vi "StandAloneTransient_TestBenchParametersArrayCreation.vi"(0 "Input Voltage Array":string[](array[string]), 1 "Board Number":string, 2 "DUT":string, 3 "Nominal Current (A)":string, 4 "XINC":string, 5 "Test Type":string, 6 "Effective LET":string, 7 "Sample Rate (SPS)":string, 9 "Threshold Percentage (%)":string, 10 "Ion (ex. Kr)":string, 11 "wfm info single capture":T1(array[cluster]), 12 "Channel":string, 13 "Mitigation Information":cluster{bool, string}) -> (14 "Array":string[][](array[string]))   [LabVIEW 2019]
uses:
  <vilib>/regexp/Match Regular Expression.xnode
panel:
  out "appended array":string[](array[string])
  out "Input Voltage Array 2":string[](array[string])
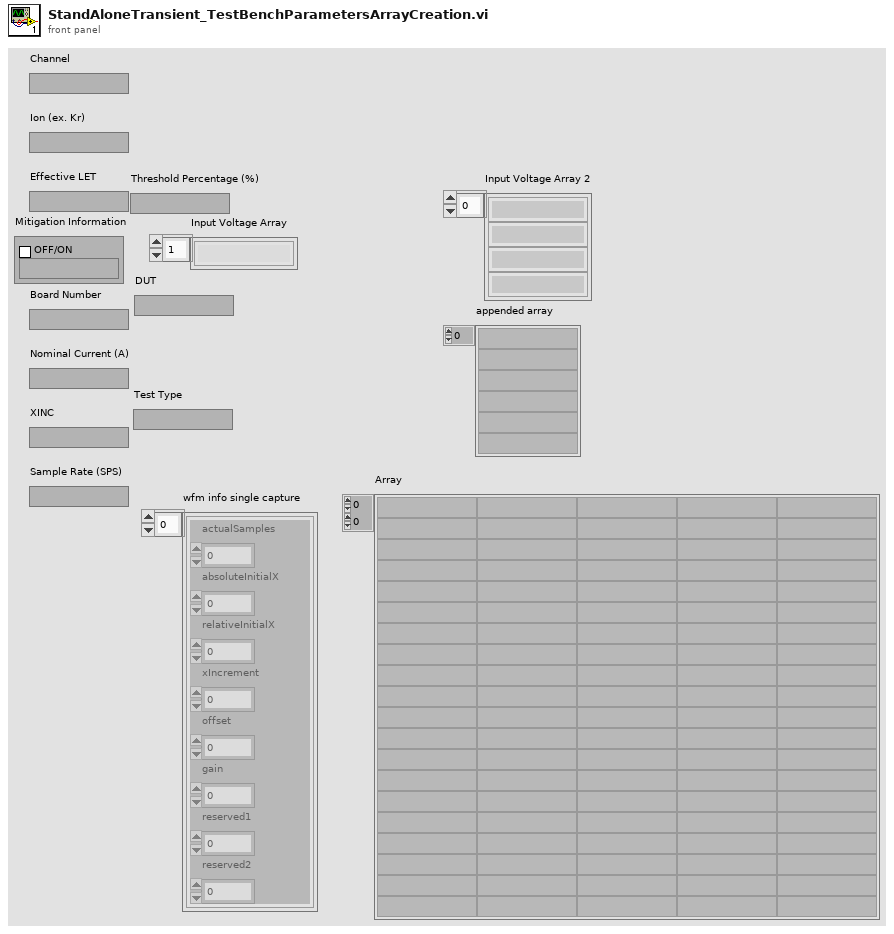
[diagram p1: front panel]
types:
  T1 = cluster{"actualSamples":i32, "absoluteInitialX":dbl, "relativeInitialX":dbl, "xIncrement":dbl, "offset":dbl, "gain":dbl, "reserved1":dbl, "reserved2":dbl}[]
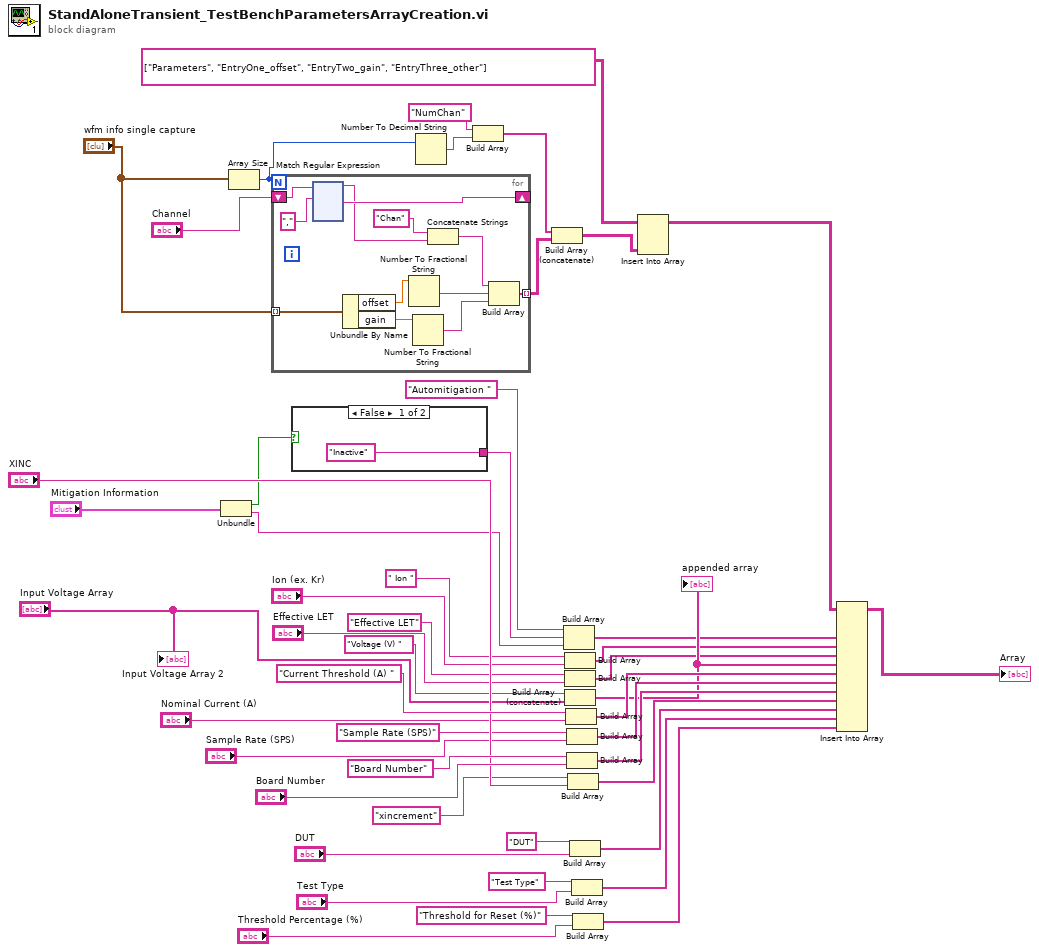
[diagram p0: block diagram]
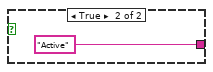
[diagram p2: hidden frame]
diagram:
  n1 = Unbundle("Mitigation Information") -> (w2:bool, w1:string)
  n2 = Array Size(array="wfm info single capture") -> (size(s)=w13:i32)
  n3 = for {
    N: w13 -> [_]
    tunnel: "wfm info single capture" -> [w59] mode=indexing
    tunnel: [w54] -> w10 mode=indexing
    shift-right: [w52] -> _
    shift-left: "Channel" -> [w53]
    n4 = xnode "Match Regular Expression"("input string"=w53, "regular expression"=",") -> ("before match"=w50:string, "after match"=w52:string)  [unwired: 4 in, 3 out]
    n5 = Unbundle By Name(w59) -> ("offset"=w57:dbl, "gain"=w58:dbl)
    n6 = Number To Fractional String(number=w57) -> (F-format string=w55:string)  [unwired: 3 in]
    n7 = Number To Fractional String(number=w58) -> (F-format string=w56:string)  [unwired: 3 in]
    n8 = Concatenate Strings("Chan" ("element"), w50) -> (w49:string)
    n9 = Build Array(w49, w55, w56) -> (w54:string[])
  }
  n10 = case shown="False" w2 {
    tunnel: ["Inactive" "Active"] -> w27
    frame False {
    }
    frame True {
    }
  }
  n11 = Number To Decimal String(number=w13) -> (decimal integer string=w12:string)  [unwired: 1 in]
  n12 = Build Array("NumChan", w12) -> (w11:string[])
  n13 = Build Array (concatenate)(w11, w10) -> (w6:string[][])
  n14 = Build Array("Automitigation " ("string"), w27, w1) -> (w25:string[])
  n15 = Build Array(" Ion " ("string"), "Ion (ex. Kr)") -> (w30:string[])
  n16 = Build Array("Effective LET" ("string"), "Effective LET") -> (w34:string[])
  n17 = Build Array (concatenate)("Voltage (V) " ("string"), "Input Voltage Array") -> (w38:string[])
  "appended array" <- w38
  n18 = Build Array("Current Threshold (A) " ("string"), "Nominal Current (A)") -> (w39:string[])
  n19 = Build Array("Sample Rate (SPS)" ("string"), "Sample Rate (SPS)") -> (w40:string[])
  n20 = Build Array("Board Number" ("string"), "Board Number") -> (w44:string[])
  n21 = Build Array("xincrement" ("string"), "XINC") -> (w43:string[])
  n22 = Build Array("DUT" ("string"), "DUT") -> (w21:string[])
  n23 = Build Array("Test Type" ("string"), "Test Type") -> (w20:string[])
  n24 = Build Array("Threshold for Reset (%)" ("string"), "Threshold Percentage (%)") -> (w15:string[])
  n25 = Insert Into Array(array=string[][] [["Parameters", "EntryOne_offset", "EntryTwo_gain", "EntryThree_other"]] ("new element/subarray"), new element=w6) -> (w5:string[][])  [unwired: 2 in]
  n26 = Insert Into Array(array=w5, new element #1=w25, new element #2=w30, new element #3=w34, new element #4=w38, new element #5=w39, new element #6=w40, new element #7=w44, new element #8=w43, new element #9=w21, new element #10=w20, new element #11=w15) -> (→"Array":string[][])  [unwired: 2 in]
  "Input Voltage Array 2" <- "Input Voltage Array"
